vi "Display-GFV.vi"(8 "error in (no error)":errorcluster, 10 "Data in":variant, 11 "?":T2=enum."Insert Image Ref For Display") -> (0 "error out":errorcluster, 2 "Image Out":T1(plugin-control), 3 "Data out":variant)   [LabVIEW 2013]
doc: "Use this template to build a VI to use as a subVI."
uses:
  DisplayGFVEnum.ctl
  DisplayDB.ctl
  <vilib>/vision/Image Controls.llb/IMAQ Image.ctl
  DbEnum.ctl
  DropletDB.ctl
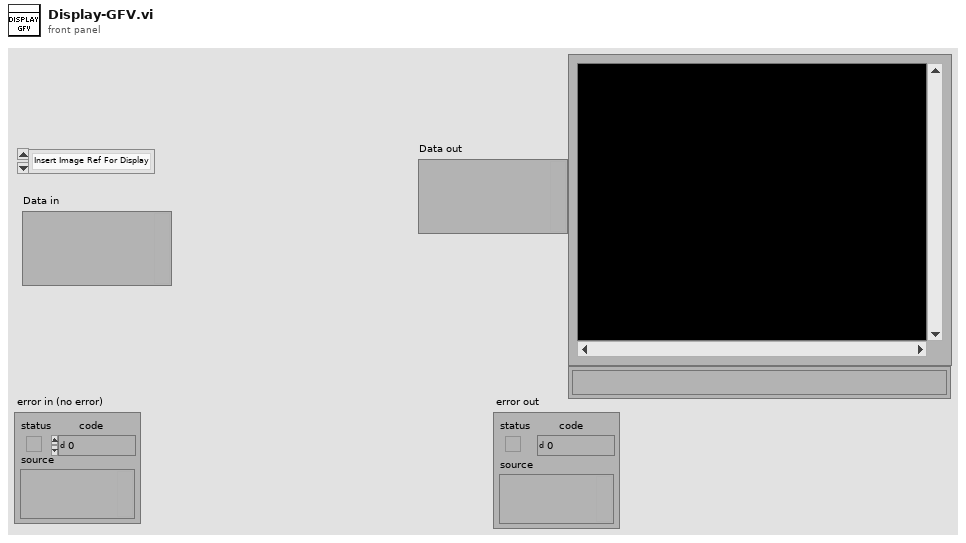
[diagram p1: front panel]
types:
  T1 = typedef "IMAQ Image.ctl" = refnum<image>
  T2 = typedef "DisplayGFVEnum.ctl" = enum16{"Update Display", "Get Image Ref for Analysis", "Insert Image Ref For Analysis", "Insert Image Ref For Display", "Init Display", "Stop Display", "Get Image Ref for Display"}
  T3 = typedef "DropletDB.ctl" = cluster{"ImageFreezeIndex":i32, "DropIndex":i32, "Position":cluster{"x":sgl, "y":sgl}, "Bounding Box":cluster{"x":sgl, "y":sgl}[], "Score":sgl, "GreyLevelInBoundingBox":dbl[], "GLDifference":dbl[], "Baseline level":dbl, "Peak":cluster{"Value":dbl, "Index":u32}, "Peak Onset":cluster{"Value":dbl, "Index":u32}, "FreezeFileName":string, "FreezeAbsTime":timestamp, "FreezeRelTime(sec)":u32, "FreezeTemperature":dbl, "ImageIndexArray":u32[], "Freeze Point Found":bool, "Baseline std":dbl, "FreezedImageArray":cluster{"Image":u8[][]}[], "Include Droplet":bool}[]
  T4 = typedef "DbEnum.ctl" = enum16{"Init", "Insert Detection Result Data", "Insert Grey Level Result", "Insert Baseline Results", "AddFreezeImagesAtCertainDroplet", "Insert Freeze Analysis Results", "GetDropDB", "GetNoFreezedDroplets", "GetGreyLevelAndDiff", "GetGreyLevelatIndexTime", "GetDropletsBoundingBox"}
  T5 = typedef "DisplayDB.ctl" = cluster{"Image Ref":T1}
  T6 = cluster{"Array[0]":i32, "Array[1]":i32, "Array[2]":i32, "Array[3]":i32}
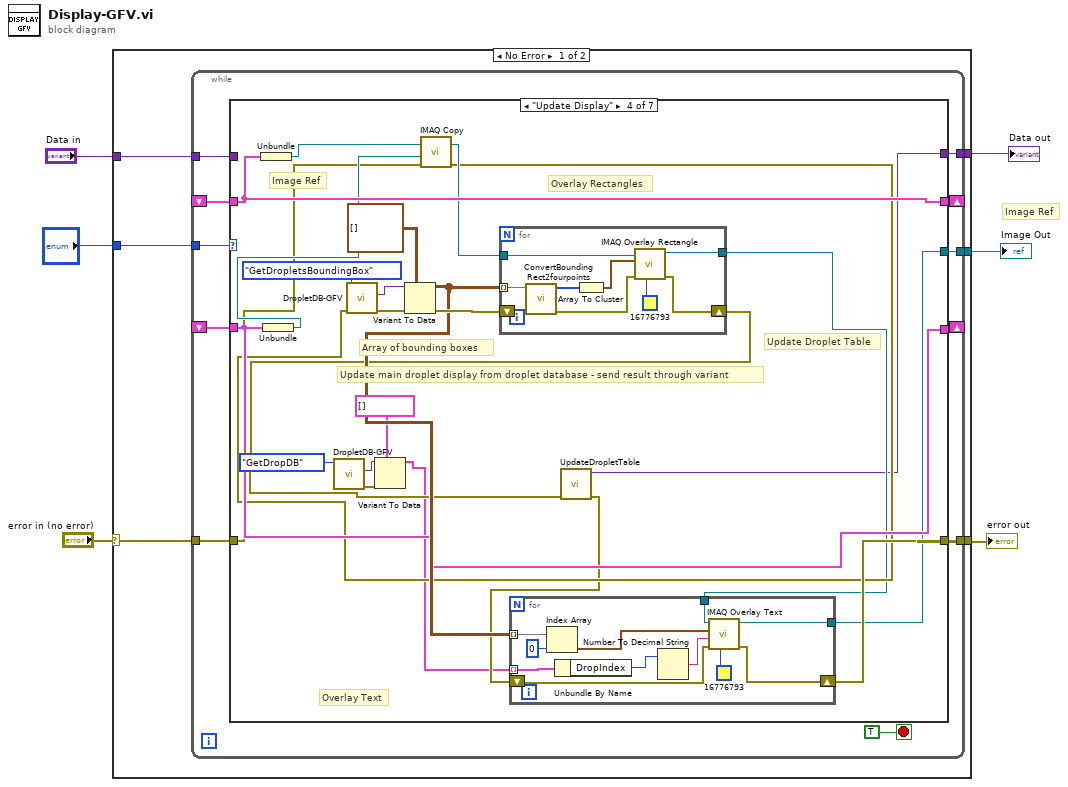
[diagram p0: block diagram]
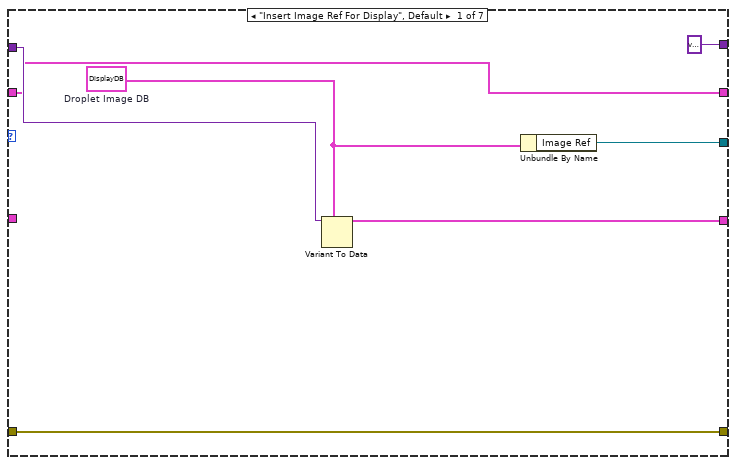
[diagram p2: hidden frame]
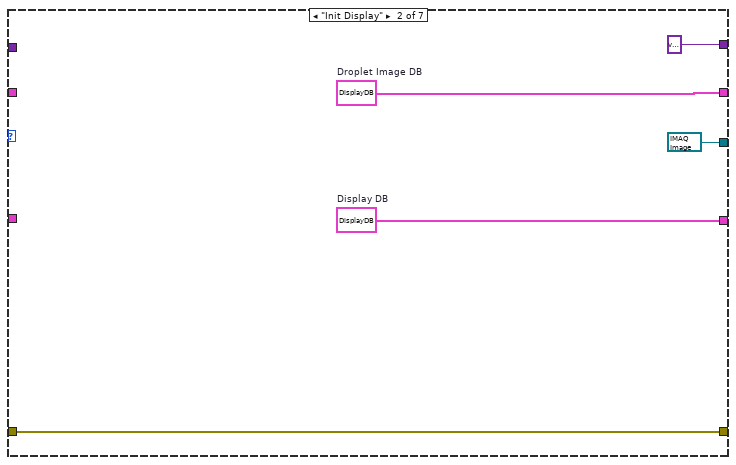
[diagram p3: hidden frame]
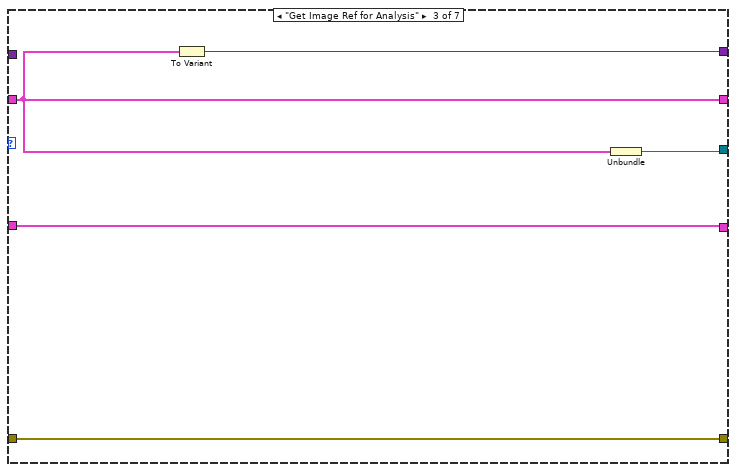
[diagram p4: hidden frame]
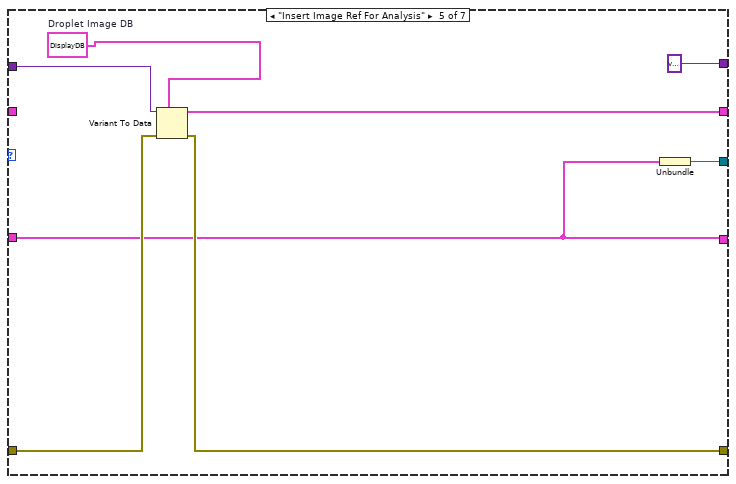
[diagram p5: hidden frame]
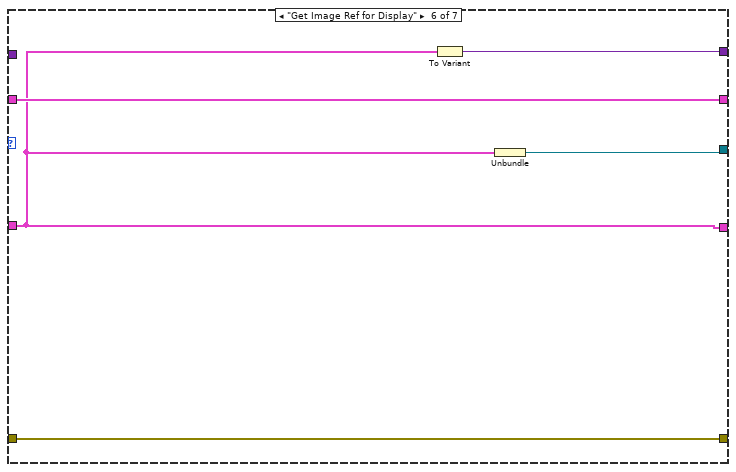
[diagram p6: hidden frame]
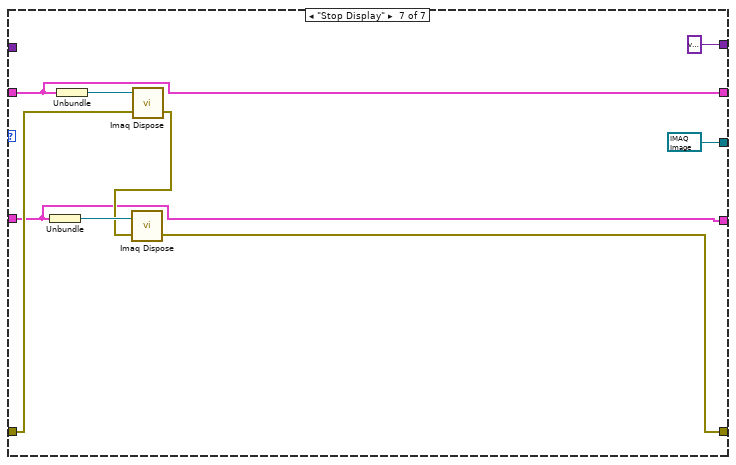
[diagram p7: hidden frame]
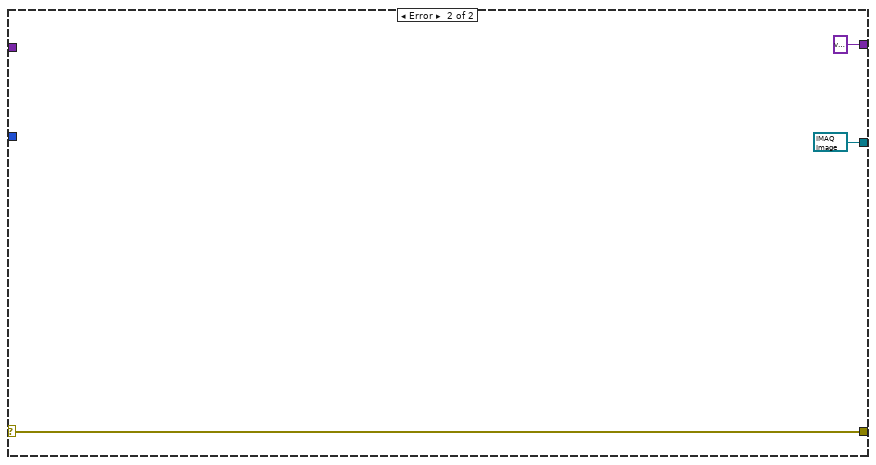
[diagram p8: hidden frame]
diagram:
  # "Image Ref"
  n1 = case shown="No Error" "error in (no error)" {
    selector: "error in (no error)" -> [w9 w109]
    tunnel: [w8 w109] -> w5
    tunnel: "?" -> [w12 _]
    tunnel: "Data in" -> [w11 _]
    tunnel: [w10 variant ("Variant")] -> w2
    tunnel: [w7 T1 refnum ("Image Out")] -> w1
    frame No Error {
      n2 = while {
        tunnel: w12 -> [w22]
        shift-right: [w21] -> _
        shift-left: _ -> [w20]
        tunnel: w11 -> [w19]
        tunnel: [w18] -> w10
        tunnel: w9 -> [w17]
        tunnel: [w16] -> w8
        tunnel: [w15] -> w7
        shift-right: [w14] -> _
        shift-left: _ -> [w13]
        stop <- TRUE stop-if-true
        n3 = case shown="\"Update Display\"" w22 {
          tunnel: [w27 w35 w36 w64 w88 w96 w99] -> w21
          tunnel: w20 -> [w27 _ w36 w64 _ w96 w99]
          tunnel: w19 -> [w30 _ _ _ w92 _ _]
          tunnel: [variant ("Variant") variant ("Variant") w40 w48 variant ("Variant") w94 variant ("Variant")] -> w18
          tunnel: w17 -> [w28 w33 w39 w52 w90 w95 w104]
          tunnel: [w28 w33 w39 w57 w89 w95 w102] -> w16
          tunnel: [w24 T1 refnum ("Image Out") w38 w49 w87 w97 T1 refnum ("Image Ref")] -> w15
          tunnel: [w29 w31 w37 w55 w86 w93 w98] -> w14
          tunnel: w13 -> [_ _ w37 w55 w86 w93 w98]
          frame "Insert Image Ref For Display", Default {
            w25 = T5 {"Image Ref"=refnum}  # Droplet Image DB
            n4 = Variant To Data(type=w25, Variant=w30) -> (data=w29:T5)  [unwired: 1 in, 1 out]
            n5 = Unbundle By Name(w25) -> ("Image Ref"=w24:T1)
          }
          frame "Init Display" {
            w31 = T5 {"Image Ref"=refnum}  # Display DB
            w35 = T5 {"Image Ref"=refnum}  # Droplet Image DB
          }
          frame "Get Image Ref for Analysis" {
            n6 = To Variant(anything=w36) -> (Variant=w40:variant)
            n7 = Unbundle(w36) -> ("Image Ref"=w38:T1)
          }
          frame "Update Display" {
            # "Update Droplet Table"
            # "Overlay Text"
            # "Overlay Rectangles"
            # "Update main droplet display from droplet database - send result through variant"
            # "Array of bounding boxes"
            # "Image Ref"
            n8 = Unbundle(w64) -> ("Image Ref"=w56:T1)
            n9 = Unbundle(w55) -> ("Image Ref"=w54:T1)
            n10 = call "DropletDB-GFV.vi"("Command In"=DbEnum."GetDropDB") -> ("error out"=w43:errorcluster, "Data out"=w42:variant)  [unwired: 9 in]
            n11 = Variant To Data(error in=w43, type=T3 [] ("DropletArray"), Variant=w42) -> (data=w41:T3)  [unwired: 1 out]
            n12 = call "IMAQ Copy"("error in (no error)"=w52, "Image Dst"=w54, "Image Src"=w56) -> ("error out"=w51:errorcluster, "Image Dst Out"=w53:T1)  [unwired: 3 in]
            n13 = call "DropletDB-GFV.vi"("error in (no error)"=w51, "Command In"=DbEnum."GetDropletsBoundingBox") -> ("error out"=w62:errorcluster, "Data out"=w63:variant)  [unwired: 8 in]
            n14 = Variant To Data(error in=w62, type=cluster{"x":sgl, "y":sgl}[][] [] ("Bounding Box"), Variant=w63) -> (data=w58:cluster{"x":sgl, "y":sgl}[][], error out=w59:errorcluster)
            n15 = for {
              tunnel: w58 -> [w84] mode=indexing
              shift-right: [w78] -> w47
              shift-left: w59 -> [w83]
              tunnel: w53 -> [w82]
              tunnel: [w76] -> w50
              n16 = call "ConvertBoundingRect2fourpoints.vi"("Error In"=w83, "Bounding Box"=w84) -> ("Error Out"=w79:errorcluster, "Array"=w80:i32[])  [unwired: 8 in]
              n17 = Array To Cluster(array=w80) -> (cluster=w81:T6)
              n18 = call "IMAQ Overlay Rectangle"("Color"=u32 16776793, "error in (no error)"=w79, "Rectangle"=w81, "Image"=w82) -> ("error out"=w78:errorcluster, "Image Out"=w76:T1)  [unwired: 6 in]
            }
            n19 = call "UpdateDropletTable.vi"("error in (no error)"=w47) -> ("error out"=w46:errorcluster, "DropletTabeVariant"=w48:variant)  [unwired: 9 in]
            n20 = for {
              tunnel: w58 -> [w72] mode=indexing
              shift-right: [w75] -> w57
              shift-left: w46 -> [w66]
              tunnel: [w73] -> w49
              tunnel: w41 -> [w69] mode=indexing
              tunnel: w50 -> [w65]
              n21 = Index Array(array=w72, index=0) -> (element=w70:cluster{"x":sgl, "y":sgl})
              n22 = Unbundle By Name(w69) -> ("DropIndex"=w67:i32)
              n23 = Number To Decimal String(number=w67) -> (decimal integer string=w68:string)  [unwired: 1 in]
              n24 = call "IMAQ Overlay Text"("Text Color (black)"=u32 16776793 ("Color"), "error in (no error)"=w66, "String"=w68, "Origin"=w70, "Image"=w65) -> ("error out"=w75:errorcluster, "Image Out"=w73:T1)  [unwired: 5 in]
            }
          }
          frame "Insert Image Ref For Analysis" {
            w85 = T5 {"Image Ref"=refnum}  # Droplet Image DB
            n25 = Variant To Data(error in=w90, type=w85, Variant=w92) -> (data=w88:T5, error out=w89:errorcluster)
            n26 = Unbundle(w86) -> ("Image Ref"=w87:T1)
          }
          frame "Get Image Ref for Display" {
            n27 = To Variant(anything=w93) -> (Variant=w94:variant)
            n28 = Unbundle(w93) -> ("Image Ref"=w97:T1)
          }
          frame "Stop Display" {
            n29 = Unbundle(w98) -> ("Image Ref"=w105:T1)
            n30 = Unbundle(w99) -> ("Image Ref"=w106:T1)
            n31 = call "Imaq Dispose"("Image"=w106, "error in (no error)"=w104) -> ("error out"=w103:errorcluster)  [unwired: 4 in]
            n32 = call "Imaq Dispose"("Image"=w105, "error in (no error)"=w103) -> ("error out"=w102:errorcluster)  [unwired: 4 in]
          }
        }
      }
    }
    frame Error {
    }
  }
  "error out" <- w5
  "Data out" <- w2
  "Image Out" <- w1
